vi "MISC Create Directory Path.vi"(0 "Path":path, 11 "Error In (no error)":errorcluster, 12 "Input Type (T:Directories only)":bool=TRUE) -> (4 "Directory Exists":bool, 6 "File Exists":bool, 15 "Error Out":errorcluster)   [LabVIEW 2017]
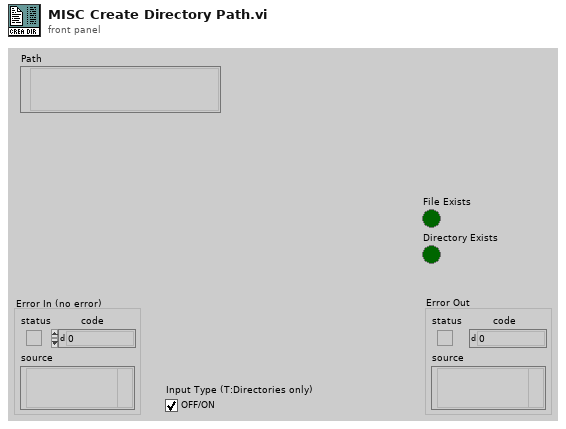
[diagram p1: front panel]
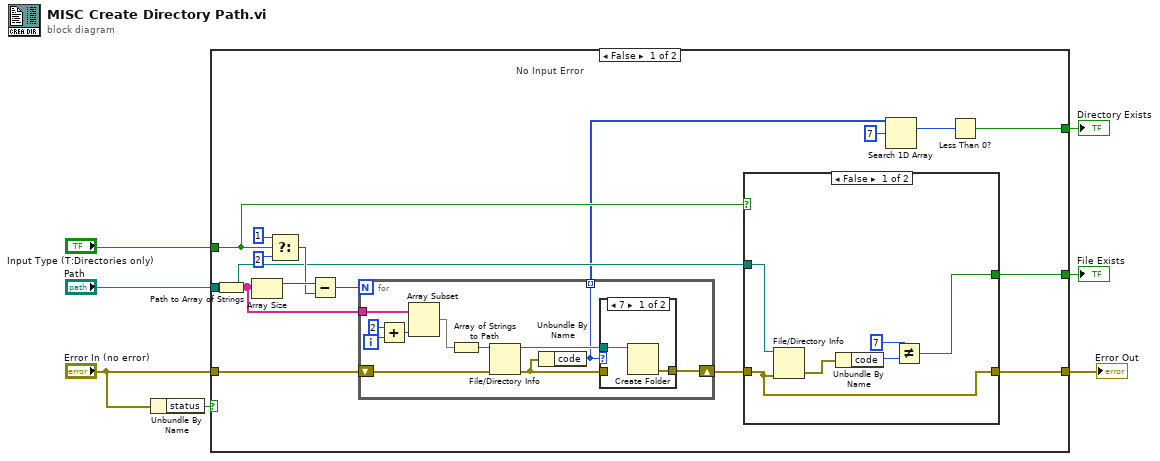
[diagram p0: block diagram]
diagram:
  n1 = Unbundle By Name("Error In (no error)") -> ("status"=w7:bool)
  n2 = case shown="False" w7 {
    tunnel: [w14 w45] -> w6
    tunnel: "Error In (no error)" -> [w21 w45]
    tunnel: "Path" -> [w13 _]
    tunnel: "Input Type (T:Directories only)" -> [w16 _]
    tunnel: [w12 _] -> w2
    tunnel: [w8 _] -> w1
    frame False {
      # "No Input Error"
      n3 = Path to Array of Strings(0:w13) -> (2:w22:string[])  [unwired: 1 out]
      n4 = Array Size(array=w22) -> (size(s)=w20:i32)
      n5 = Select(t=1 ("y"), s=w16, f=2 ("y")) -> (s? t:f=w17:i32)
      n6 = Subtract(x=w20, y=w17) -> (x-y=w23:i32)
      n7 = for {
        N: w23 -> [_]
        shift-right: [w39] -> w15
        shift-left: w21 -> [w41]
        tunnel: w22 -> [w37]
        tunnel: [w31] -> w11 mode=indexing
        i -> [w36]
        n8 = Add(x=2, y=w36) -> (x+y=w35:i32)
        n9 = Array Subset(array=w37, length=w35) -> (w34:string[])  [unwired: 1 in]
        n10 = Array of Strings to Path(0:w34) -> (2:w33:path)  [unwired: 1 out]
        n11 = File/Directory Info(path=w33, error in=w41) -> (path out=w38:path, error out=w40:errorcluster)  [unwired: 5 out]
        n12 = Unbundle By Name(w40) -> ("code"=w31:i32)
        n13 = case shown="7" w31 {
          tunnel: w40 -> [_ w44]
          tunnel: [w43 w44] -> w39
          tunnel: w38 -> [w42 _]
          frame 7 {
            n14 = Create Folder(path (use dialog)=w42) -> (error out=w43:errorcluster)  [unwired: 1 in, 3 out]
          }
          frame Default {
          }
        }
      }
      n15 = case shown="False" w16 {
        tunnel: w15 -> [w27 w30]
        tunnel: [w27 w30] -> w14
        tunnel: w13 -> [w29 _]
        tunnel: [w24 _] -> w12
        frame False {
          n16 = File/Directory Info(path=w29, error in=w27) -> (error out=w28:errorcluster)  [unwired: 6 out]
          n17 = Unbundle By Name(w28) -> ("code"=w26:i32)
          n18 = Not Equal?(x=7, y=w26) -> (x != y?=w24:bool)
        }
        frame True {
        }
      }
      n19 = Search 1D Array(1D array=w11, element=7) -> (index of element=w9:i32)  [unwired: 1 out]
      n20 = Less Than 0?(x=w9) -> (x < 0?=w8:bool)
    }
    frame True {
      # "Input Error"
    }
  }
  "Error Out" <- w6
  "File Exists" <- w2
  "Directory Exists" <- w1
